vi "Stop Core.vi"(10 "final error code":i32, 11 "MonitoredMediator in":refnum<class "MonitoredMediator.lvclass">) -> (3 "MonitoredMediator out":refnum<class "MonitoredMediator.lvclass">)   [LabVIEW 2018, in "MVA Framework.lvlib" / "MonitoredMediator.lvlib" / "MonitoredMediator.lvclass"]
doc: "(<B>Filename</B>: Actor Framework.lvlib:Actor.lvclass:Stop Core.vi)\n\nDefines what the actor does before it stops. Use the <B>final error code</B> input to determine whether the actor shut down in response to an error.\n\nBy default, this method does nothing. A descendant class may override it to define behavior, such as shutting down any processes the actor initiated in its override of the Actor Core method."
uses:
  MonitoredMediator.lvclass
  Mediator/Mediator/Mediator.lvclass
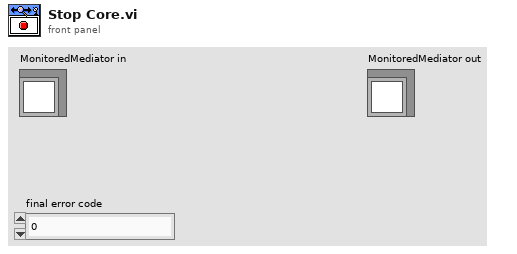
[diagram p1: front panel]
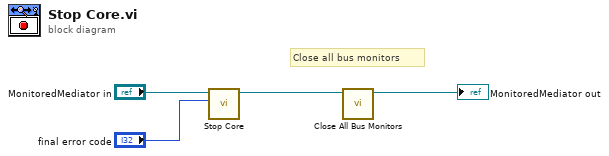
[diagram p0: block diagram]
diagram:
  # "Close all bus monitors"
  n1 = call-parent "Stop Core.vi"("final error code"="final error code", "Mediator in"="MonitoredMediator in") -> ("Mediator out"=w2:refnum<class "MonitoredMediator.lvclass">)  [unwired: 9 in]
  n2 = call "Close All Bus Monitors.vi"("MonitoredMediator in"=w2) -> ("MonitoredMediator out"=→"MonitoredMediator out":refnum<class "MonitoredMediator.lvclass">)  [unwired: 10 in]
